vi "creat array.vi"(1 "size":i32) -> (0 "array":i32[](array[numeric]))   [LabVIEW 2010]
doc: "按输入参数n构建一个整型数组。数组元素个数等于2n-1,数组元素值为1,2,3...n...3,2,1。"
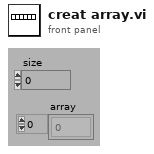
[diagram p1: front panel]
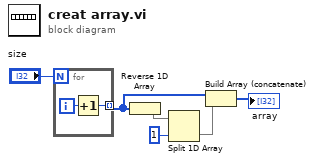
[diagram p0: block diagram]
diagram:
  n1 = for {
    N: "size" -> [_]
    tunnel: [w7] -> w4 mode=indexing
    i -> [w8]
    n2 = Increment(x=w8) -> (x+1=w7:i32)
  }
  n3 = Reverse 1D Array(array=w4) -> (reversed array=w3:i32[])
  n4 = Split 1D Array(array=w3, index=1) -> (second subarray=w1:i32[])  [unwired: 1 out]
  n5 = Build Array (concatenate)(w4, w1) -> (→"array":i32[])
